vi "global-csm-ini-db-change-flag.vi"() -> ()   [LabVIEW 2017, in "INI-Static-Variable-Support.lvlib"]
uses:
  INI-Static-Variable-Support.lvlib
panel:
  in  "csm-ini-db-change-flag":u64=18446744073709551615 format="%x"
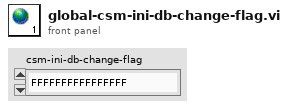
[diagram p1: front panel]
diagram:
